vi "SR430_close.vi"(0 "SR430 VISA Cluster":T1, 11 "error in (no error)":errorcluster) -> (15 "error out":errorcluster)   [LabVIEW 2015, in "SR430Driver.lvlib"]
doc: "This VI closes the I/O interface with the instrument.\n\nCopyright (C) \nGesellschaft f. Schwerionenforschung, GSI\nPlanckstr. 1\n64291 Darmstadt\nGermany\n\nContact: http://www-wnt.gsi.de/labview, d.beck@gsi.de\n\nThis program is free software; you can redistribute it and/or\nmodify it under the terms of the GNU General Public License\nas published by the Free Software Foundation; either version 2\nof the License, or (at your option) any later version.\n\nThis program is distributed in the hope that it will be useful,\nbut WITHOUT ANY WARRANTY; without even the implied warranty of\nMERCHANTABILITY or FITNESS FOR A PARTICULAR PURPOSE. See the\nGNU General Public License for more details (http://www.gnu.org)."
uses:
  SR430Driver.lvlib
  SR430_VISA Control.ctl
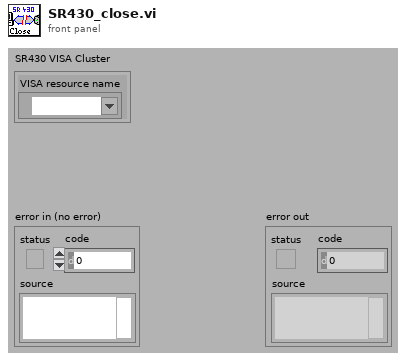
[diagram p1: front panel]
types:
  T1 = typedef "SR430Driver.lvlib/SR430_VISA Control.ctl" = cluster{"VISA resource name":refnum<visa-resource-name>}
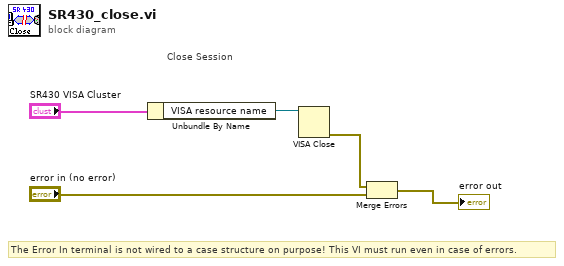
[diagram p0: block diagram]
diagram:
  # "The Error In terminal is not wired to a case structure on purpose! This VI must run even in case of errors."
  # "Close Session"
  n1 = Unbundle By Name("SR430 VISA Cluster") -> ("VISA resource name"=w2:refnum<visa-resource-name>)
  n2 = VISA Close(VISA resource name=w2) -> (error out=w1:errorcluster)  [unwired: 1 in]
  n3 = Merge Errors(w1, "error in (no error)") -> (→"error out":errorcluster)
